vi "Example_Get Instrument ID.vi"() -> ()   [LabVIEW 2011]
panel:
  in  "Ethernet":T1={"Port"=10001, "Timeout"=1000, "IP Address"=""}
  in  "Remote Mode":u16(ring) items=["USB", "RS232", "GPIB", "Ethernet"]
  in  "Baud Rate (921600)":u32=921600
  out "Read Buffer":string
  out "Error out":errorcluster caption="error out"
  in  "error in (no error)":errorcluster
  in  "VISA resource name":refnum<visa-resource-name>
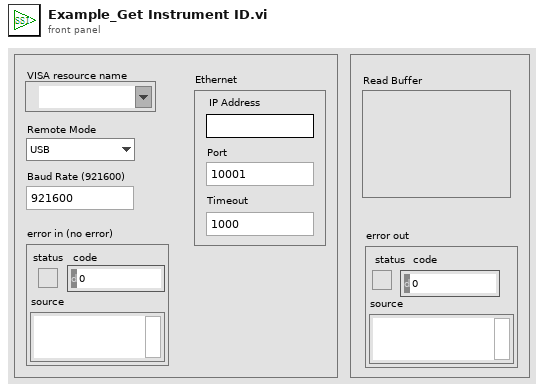
[diagram p1: front panel]
types:
  T1 = cluster{"Port":u32, "Timeout":u32, "IP Address":string}
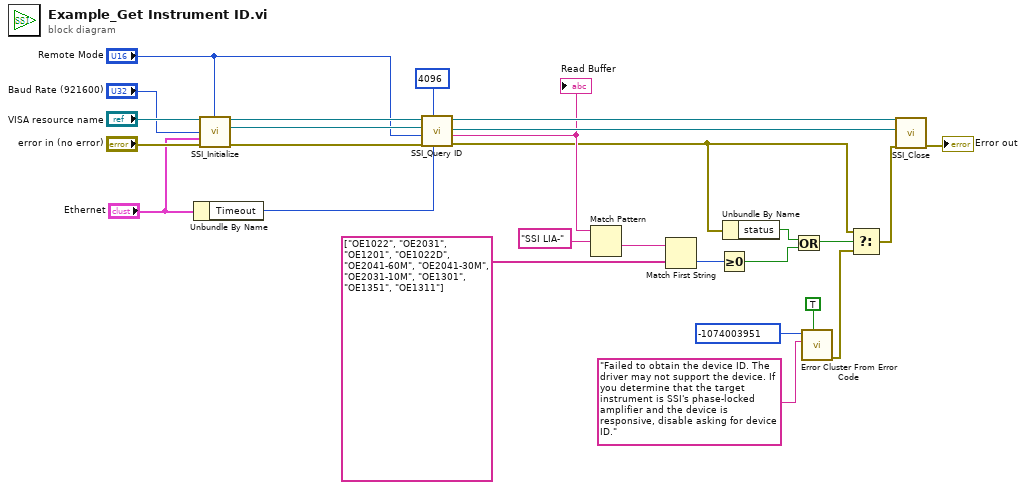
[diagram p0: block diagram]
diagram:
  n1 = Unbundle By Name("Ethernet") -> ("Timeout"=w1:u32)
  n2 = call "SSI_Initialize.vi"("VISA resource name"="VISA resource name", "Remote Mode"="Remote Mode", "baud rate (921600)"="Baud Rate (921600)", "Ethernet"="Ethernet", "error in (no error)"="error in (no error)") -> ("VISA resource name out"=w12:refnum<visa-resource-name>, "connection ID(Ethernet)"=w10:refnum<k5>, "error out"=w11:errorcluster)  [unwired: 8 in]
  n3 = call "SSI_Query ID.vi"("Timeout"=w1, "Number of bytes"=u32 4096, "Error in (no error)"=w11, "Remote Mode"="Remote Mode", "Connection ID in"=w10, "VISA resource name"=w12) -> ("Error out"=w5:errorcluster, "Read Buffer"=w6:string, "Connection ID out"=w8:refnum<k5>, "VISA resource  out"=w9:refnum<visa-resource-name>)  [unwired: 2 in]
  "Read Buffer" <- w6
  n4 = Match Pattern(string=w6, regular expression="SSI LIA-" ("正则表达式")) -> (after substring=w23:string)  [unwired: 1 in, 3 out]
  n5 = Match First String(2:string[] ["OE1022", "OE2031", "OE1201", "OE1022D", "OE2041-60M", "OE2041-30M", "OE2031-10M", "OE1301", "OE1351", "OE1311"] ("string array"), 3:w23) -> (0:w24:i32)  [unwired: 1 out]
  n6 = Greater Or Equal To 0?(x=w24) -> (x >= 0?=w25:bool)
  n7 = Unbundle By Name(w5) -> ("status"=w7:bool)
  n8 = Or(x=w7, y=w25) -> (x .or. y?=w22:bool)
  n9 = call <vilib>:"Error Cluster From Error Code.vi"("show call chain? (False)"=TRUE, "error message (\"\")"="Failed to obtain the device ID. The driver may not support the device. If you determine that the target instrument is SSI's phase-locked amplifier and the device is responsive, disable asking for device ID." ("Source (VI Name)"), "error code (0)"=-1074003951 ("Code")) -> ("error out"=w18:errorcluster)  [unwired: 1 in, 5 out]
  n10 = Select(t=w5, s=w22, f=w18) -> (s? t:f=w13:errorcluster)
  n11 = call "SSI_Close.vi"("Error in (no error)"=w13, "Connection ID in"=w8, "VISA resource name"=w9) -> ("Error out"=→"Error out":errorcluster)  [unwired: 4 in]
